vi "문자열 읽기.vi"() -> ()   [LabVIEW 2014]
panel:
  out "배열":dbl[][](array[numeric])
  out "텍스트":string
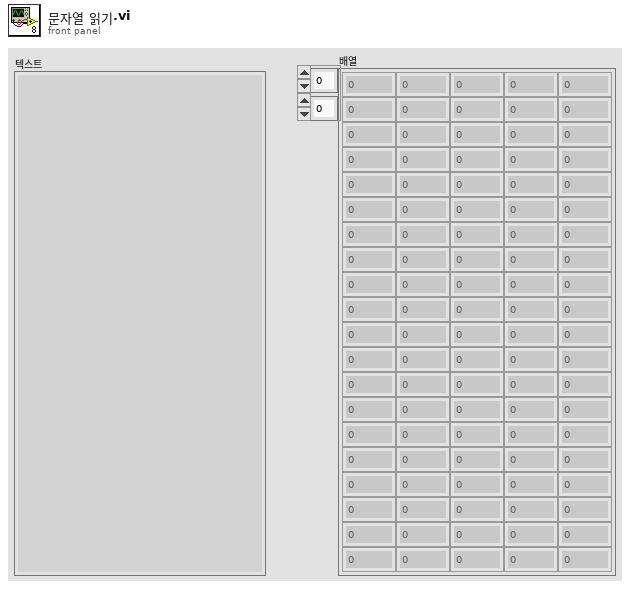
[diagram p1: front panel]
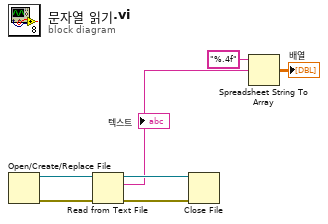
[diagram p0: block diagram]
diagram:
  n1 = Open/Create/Replace File() -> (refnum out=w7:refnum<file>, error out=w5:errorcluster)  [unwired: 6 in, 1 out]
  n2 = Read from Text File(file (use dialog)=w7, error in=w5) -> (refnum out=w6:refnum<file>, text=w3:string, error out=w4:errorcluster)  [unwired: 2 in, 1 out]
  "텍스트" <- w3
  n3 = Close File(refnum=w6, error in=w4) -> ()  [unwired: 2 out]
  n4 = Spreadsheet String To Array(format string="%.4f" ("포맷 문자열"), spreadsheet string=w3) -> (array=→"배열":dbl[][])  [unwired: 2 in]
